vi "BotSpeak_Error.vi"(0 "Error String":string) -> ()   [LabVIEW 2014]
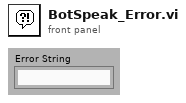
[diagram p1: front panel]
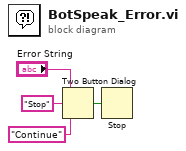
[diagram p0: block diagram]
diagram:
  n1 = Two Button Dialog(message="Error String", 1:"Continue" ("T button name (\"OK\")"), 2:"Stop" ("T button name (\"OK\")")) -> (T button?=w4:bool)
  n2 = Stop(stop? (T)=w4) -> ()
